vi "Read Refs.vi"(11 "Setup in":refnum<class "Setup.lvclass">) -> (2 "Refs":refnum<class "Refs.lvclass">)   [LabVIEW 2025, in "jettl.lvlib" / "Setup.lvlib" / "Setup.lvclass"]
uses:
  Setup.lvclass
  Refs/Refs.lvclass
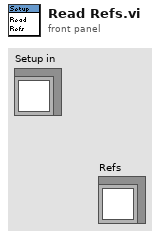
[diagram p1: front panel]
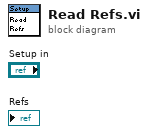
[diagram p0: block diagram]
diagram:
